vi "Dashboard Main.vi"() -> ()   [LabVIEW 2014]
uses:
  <vilib>/event_ctls.llb/eventvkey.ctl
  <vilib>/Rock Robotics/WPI/Dashboard/WPI_DashboardLogging Global.vi
  <vilib>/Rock Robotics/Network Tables/SD Read Number.vi
  <vilib>/Utility/config.llb/Write Key (String).vi
  <vilib>/Utility/config.llb/Write Key (I32).vi
  <vilib>/Utility/config.llb/NI_LVConfig.lvlib
panel:
  in  "TCP":refnum<k5>
  in  "Rec Mode":enum32{"Stop", "Record", "Playback"}(radio)
  in  "Vision":u16(ring) items=["Camera Off", "USB Camera SW", "USB Camera HW", "IP Camera"]
  out "Camera IP":string
  out "Image Message":string="Timeout in Camera Communications"
  in  "Dashboard Tab":T1(tab)
  in  "Camera Settings":T2={"Frame Rate"=30, "Compression"=30, "Size"=1} {"Frame Rate" scale=1.0..30.0; "Size" items=["640x480", "320x240", "160x120"]}
  out "MotorChart R":cluster{"Numeric":dbl, "Numeric":dbl}(graph)
  out "MotorChart L":T3(graph)
  out "MotorSliders R":cluster{"MotorSlide1":dbl, "MotorSlide2":dbl} {"MotorSlide2" scale=-1.0..1.0 scale format="%#_2e"; "MotorSlide1" scale=-1.0..1.0 scale format="%#_2e"}
  out "MotorSliders L":T4 {"MotorSlide4 2" scale=0.0..14.0 scale format="%#_2e"; "MotorSlide2" scale=-1.0..1.0 scale format="%#_2e"; "MotorSlide1" scale=-1.0..1.0 scale format="%#_2e"}
  out "Gyro":dbl(knob) scale=0.0..360.0
  out "JS1 Z":dbl(slide) scale=-1.0..1.0 scale format="%#_2e"
  out "JS1 Graph":cluster{"X":dbl, "Y":dbl}[](graph)
  out "JS1 Buttons":T5
  out "JS2 Z":dbl(slide) scale=-1.0..1.0 scale format="%#_2e"
  out "JS2 Graph":cluster{"X":dbl, "Y":dbl}[](graph)
  out "JS2 Buttons":T5
  out "Mode":T6(ring)=enum."Auto Disabled"
  in  "DB Camera Config":bool
  out "fps":dbl format="%#.1g"
  out "Mbps":dbl format="%#.1g"
  out "Mbps 2":bool
  in  "DB/String 9":string
  in  "DB/String 8":string
  in  "DB/String 7":string
  in  "DB/String 6":string
  in  "DB/String 5":string
  in  "DB/String 4":string
  in  "DB/String 3":string
  in  "DB/String 2":string
  in  "DB/String 1":string
  in  "DB/String 0":string
  in  "DB/Slider 0":dbl(slide) scale=0.0..5.0
  in  "DB/Slider 1":dbl(slide) scale=0.0..5.0
  in  "DB/Slider 2":dbl(slide) scale=0.0..5.0
  in  "DB/Slider 3":dbl(slide) scale=0.0..5.0
  out "DB/LED 3":bool
  out "DB/LED 2":bool
  out "DB/LED 1":bool
  out "DB/LED 0":bool
  in  "DB/Button 3":bool
  in  "DB/Button 2":bool
  in  "DB/Button 1":bool
  in  "DB/Button 0":bool caption="New Name"
  in  "Autonomous_Modes":bool[](array[boolean])
  in  "Test_Knob":u16(knob) scale=0.0..5.0
  in  "Test Slider":dbl(slide) scale=0.0..100.0 scale format="%#_3g"
  in  "On/Off":bool caption="Solenoid"
  in  "Test Name":u16(ring) items=["Select the test to run...", "Example Test", "-------------------------------", "List of tests is built in robot code.", "Replace with your own automated tests."]
  in  "Test Tree":string(tree)
  in  "Motor":cluster{"Value":dbl, "Enable":bool} {"Value" scale=-1.0..1.0 scale format="%#_3g"}
  out "Progress":T7 {"Test Progress" scale=0.0..100.0}
  in  "Rev/Fwd":cluster{"Forward":bool, "Reverse":bool}
  in  "Test Ring":u16(ring) items=["Monochrome", "Color"]
  in  "Listbox":i32(listbox)
  out "Tree":string(tree)
  out "Camera Image":T8(plugin-control)
  out "Boolean":bool
  # "Left"
  # "Front"
  # "Right"
  # "Battery"
  # "Single Tote"
  # "Double Tote"
  # "Triple Tote"
  # "Butterfly"
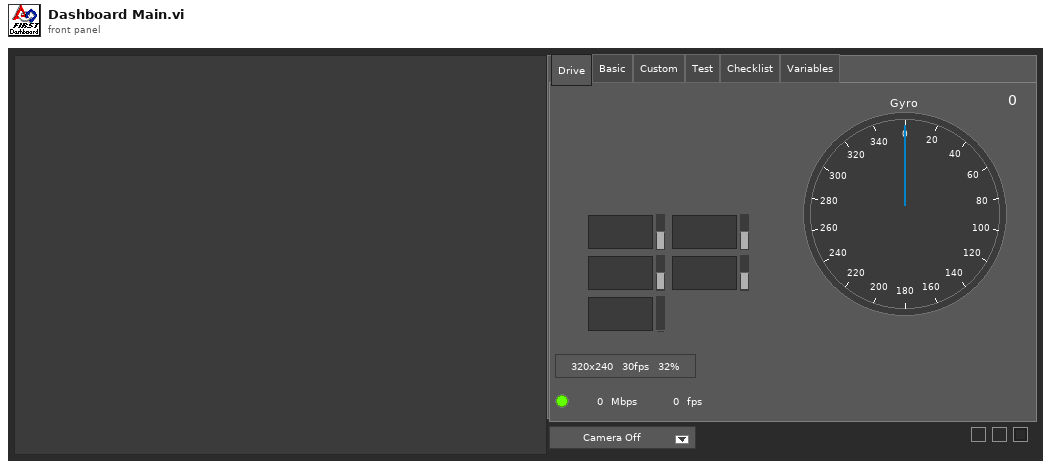
[diagram p1: front panel]
types:
  T1 = enum32{"Drive", "Basic", "Custom", "Test", "Checklist", "Variables"}
  T2 = cluster{"Frame Rate":i32, "Compression":i32, "Size":u16}
  T3 = cluster{"Numeric":dbl, "Numeric":dbl, "Battery V":dbl}
  T4 = cluster{"MotorSlide1":dbl, "MotorSlide2":dbl, "MotorSlide4 2":dbl}
  T5 = cluster{bool, bool, bool, bool, bool, bool, bool, bool, bool, bool, bool, bool}
  T6 = enum8{"Tele-Op Disabled", "Tele-Op Enabled", "Auto Disabled", "Auto Enabled", "Test Disabled", "Test Enabled", "Disconnected", "No Code", "E-Stop"}
  T7 = cluster{"Test Progress":u8, "Test Progress Text":string}
  T8 = typedef "IMAQ Image.ctl" = refnum<image>
  T9 = typedef "Image Type" = u32
  T10 = cluster{"Camera Image":refnum<vi>, "Dashboard Tab":refnum<vi>, "Boolean":refnum<vi>, "Vision":refnum<vi>, "Rec Mode":refnum<vi>, "Test Slider":refnum<vi>, "On/Off ":refnum<vi>, "Test Ring":refnum<vi>, "Rev/Fwd":refnum<vi>, "Test Name":refnum<vi>, "Motor":refnum<vi>, "Progress":refnum<vi>, "CheckList":refnum<vi>, "Tree":refnum<vi>, "Test Tree":refnum<vi>}
  T11 = cluster{"Error Strings":string, "Disable Counts":cluster{u16, u16}, "Rail Faults":cluster{u16, u16, u16}, "Robot IP":string, "DB Mode":u8, "Event Info":cluster{"Name":string, "Type":u8, "Number":u16, "Replay":u8}, "Camera Addr":string}
  T12 = cluster{"Storage":cluster{"Disk Free":u64, "RAM Block":u32, "RAM free":u32}, "CPU Utilization":cluster{"CPU % ISR":sgl, "CPU % Time Crit":sgl, "CPU % Timed Str":sgl, "CPU % High":sgl, "CPU % Above":sgl, "CPU % Normal":sgl, "CPU % Low":sgl}, "CAN":cluster{"% Bus Utilization":sgl, "Bus Off Cnt":u32, "TX_FIFO Full Cnt":u32, "Receive Error Cnt":u8, "Transmit Error Cnt":u8}, "HID":cluster{"HID Outputs":u32, "Rumble Low":u16, "Rumble High":u16}[]}
  T13 = cluster{"Status bits":cluster{"Test Mode":bool, "Autonomous":bool, "Enabled":bool, "Code Start":bool, "Brownout":bool, "Reserved 2":bool, "Reserved 3":bool, "E-Stop":bool}, "Code Trace":cluster{"Disabled":bool, "TeleOp":bool, "Auto":bool, "Test":bool}, "Controller Type":enum16{"unknown", "cRIO", "roboRio"}, "Code?":enum16{"unknown", "noCode", "code"}, "Battery V":dbl}
  T14 = cluster{"Control Bits":cluster{"TestMode":bool, "Autonomous":bool, "Enabled":bool, "FMS Present":bool, bool, bool, bool, "E-Stop":bool}, "Team Station ":u8, "Countdown":sgl, "Joystick Values":cluster{"Axes":dbl[], "Buttons":bool[], "POVs":i16[]}[]}
  T15 = cluster{"Axes":dbl[], "Buttons":bool[], "POVs":i16[]}[]
  T16 = cluster{"Axes":dbl[], "Buttons":bool[], "POVs":i16[]}
  T17 = cluster{"Buttons[0]":bool, "Buttons[1]":bool, "Buttons[2]":bool, "Buttons[3]":bool, "Buttons[4]":bool, "Buttons[5]":bool, "Buttons[6]":bool, "Buttons[7]":bool, "Buttons[8]":bool, "Buttons[9]":bool, "Buttons[10]":bool, "Buttons[11]":bool}
  T18 = typedef "NI_LVConfig.lvlib/Config Data RefNum.ctl" = refnum<k1>
  T19 = cluster{"Operation":enum16{"Update", "Clear"}, "Color Box":u32}[]
  T20 = typedef "eventvkey.ctl" = enum16{"ASCII", "Enter", "Return", "Shift", "Ctrl", "Alt", "Cmd", "Opt", "Caps", "NumLock", "Clear", "Break", "Up", "Down", "Left", "Right", "Insert", "Delete", "Home", "End", "PageUp", "PageDown", "Escape", "Help", "Pause", "ScrollLock", "F1", "F2", "F3", "F4", "F5", "F6", "F7", "F8", "F9", "F10", "F11", "F12", "F13", "F14", "F15", "F16", "F17", "F18", "F19", "F20", "F21", "F22", "F23", "F24", "Play", "VolumeUp", "VolumeDown", "Mute", "Two Byte Char"}
  T21 = cluster{"Image Size":bool, "Image Type":bool, "Pixel Value":bool, "ROI Information":bool, "Zoom Factor":bool}
  T22 = enum8{"Enabled", "Disabled", "Disabled and Grayed Out"}
  T23 = cluster{"Operation":enum16{"Update", "Clear"}, "Color Box":u32}
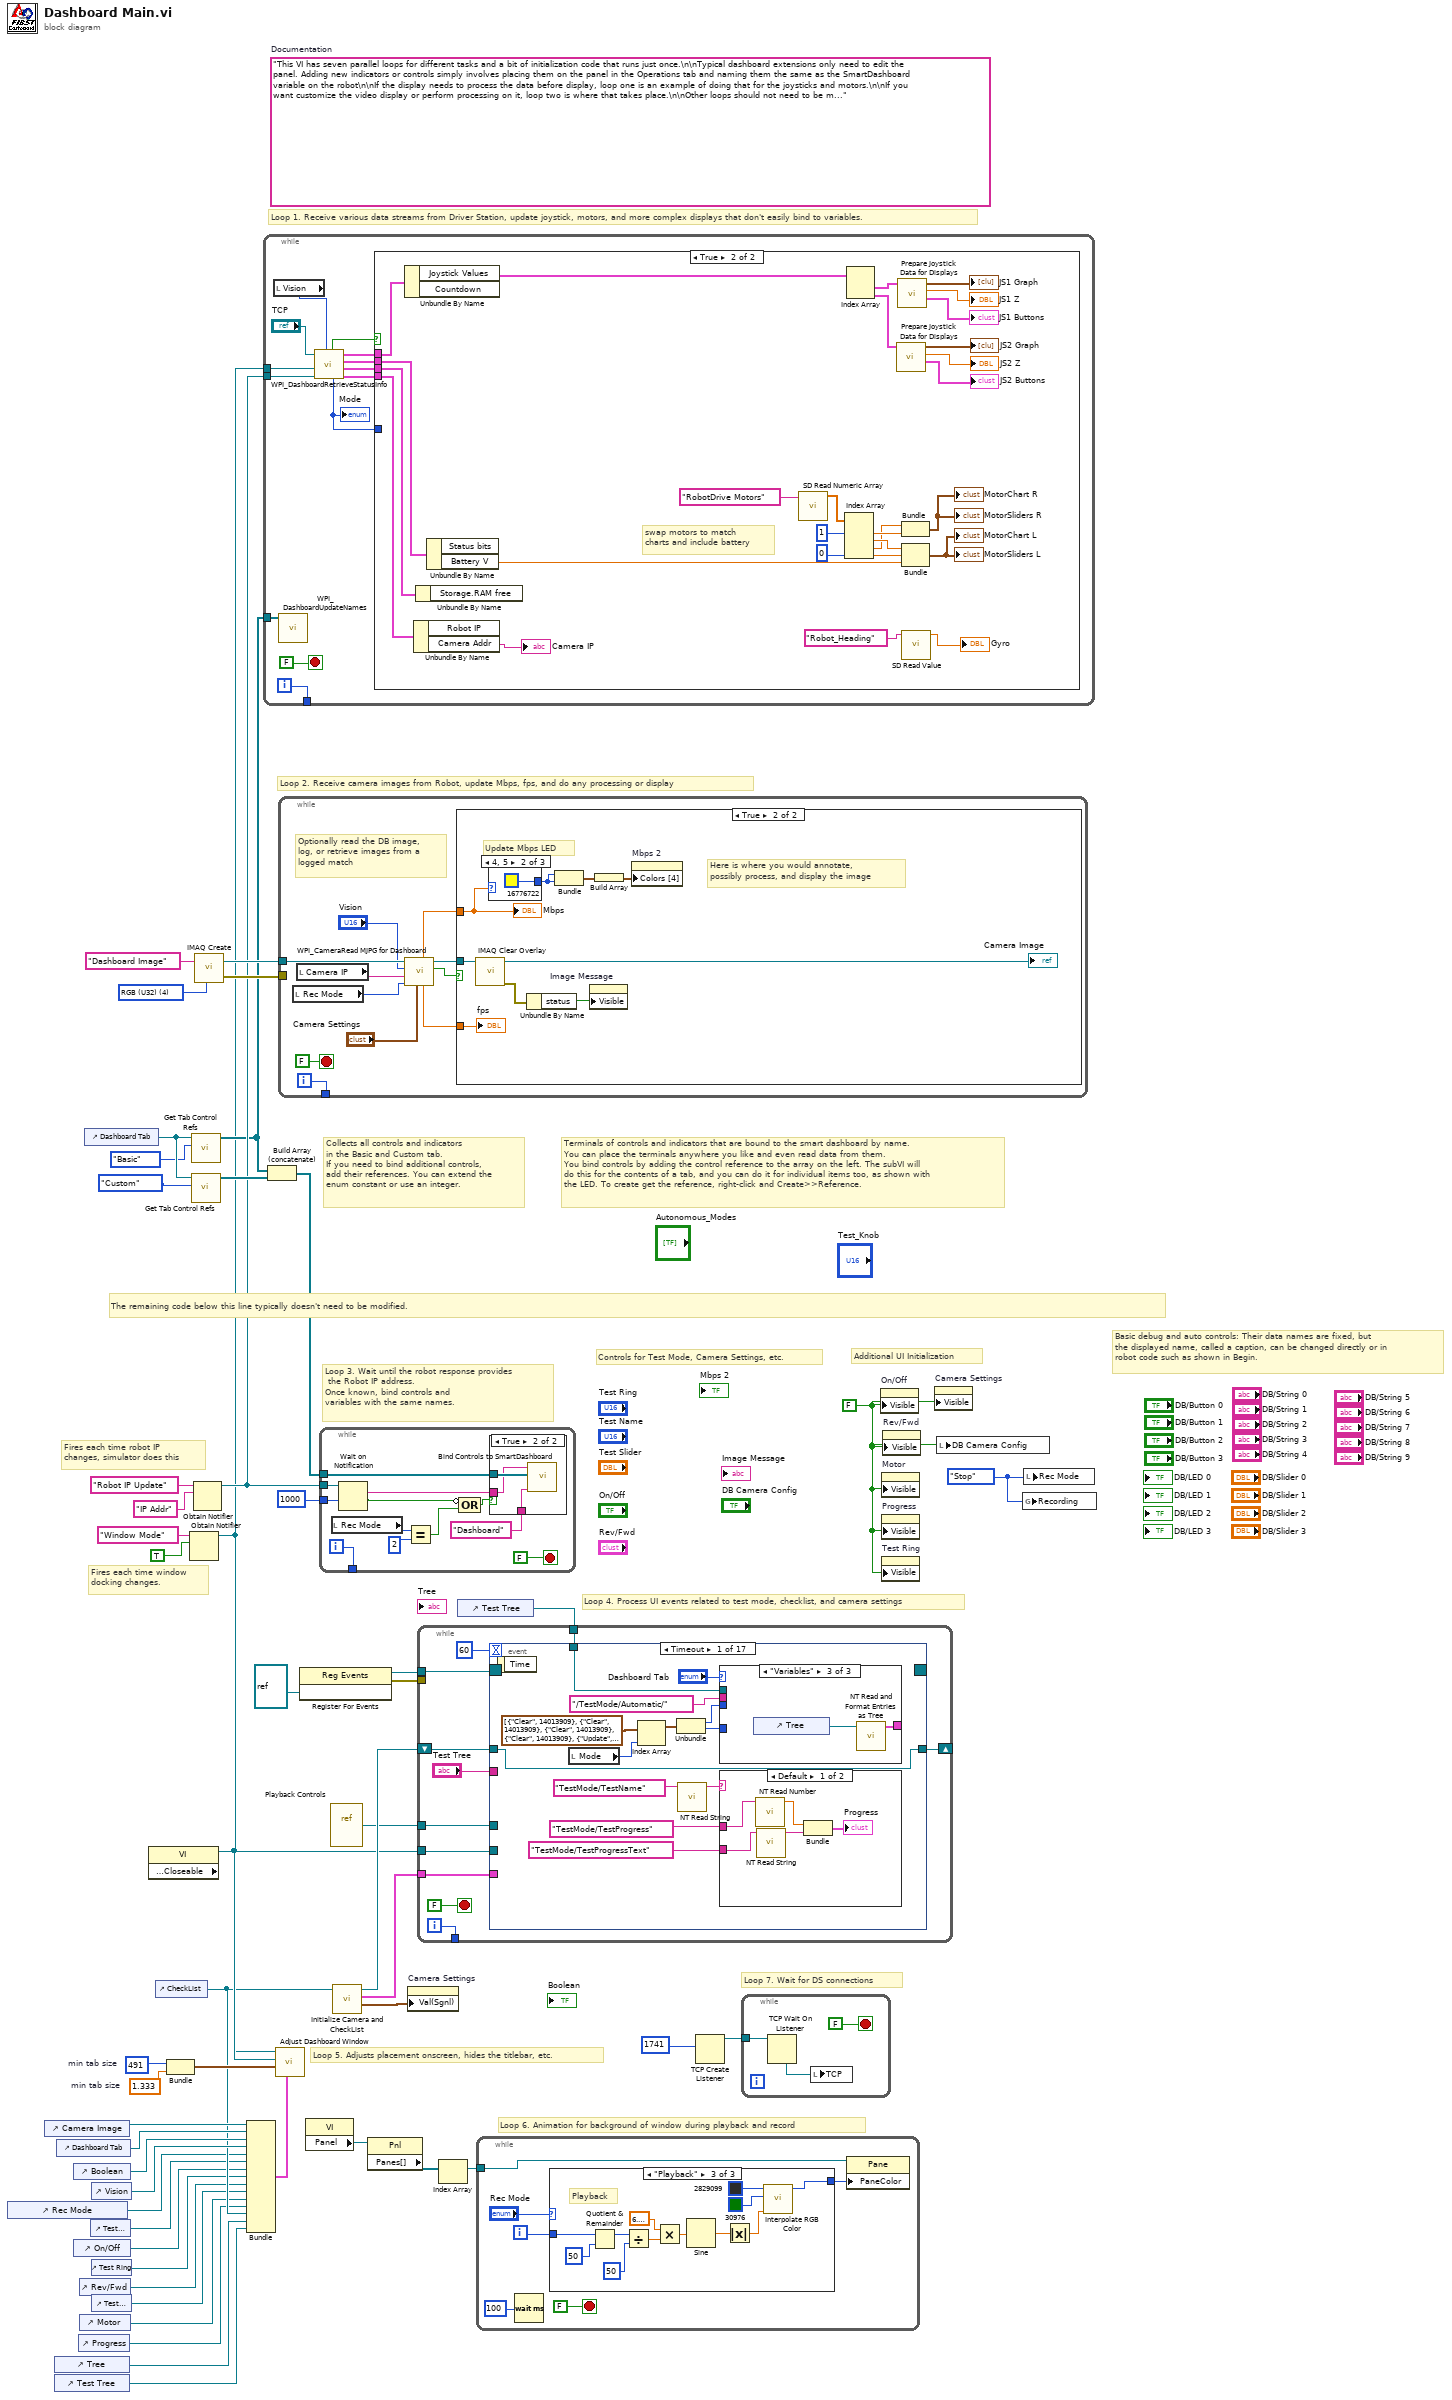
[diagram p0: block diagram]
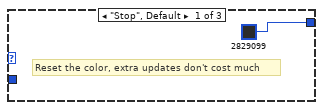
[diagram p3: hidden frame]
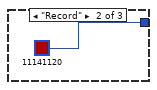
[diagram p4: hidden frame]
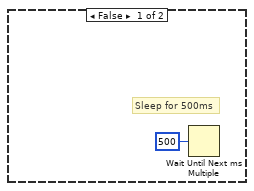
[diagram p6: hidden frame]
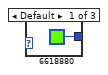
[diagram p7: hidden frame]
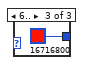
[diagram p8: hidden frame]
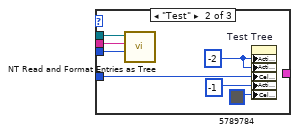
[diagram p10: hidden frame]
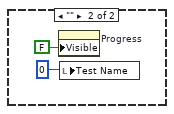
[diagram p11: hidden frame]
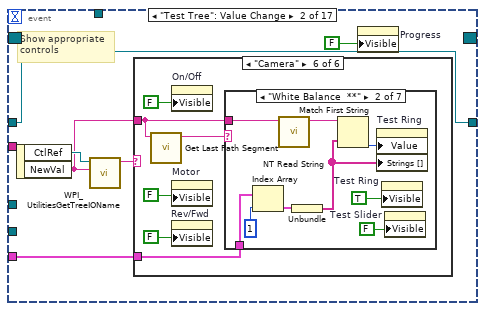
[diagram p12: hidden frame]
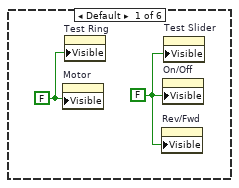
[diagram p13: hidden frame]
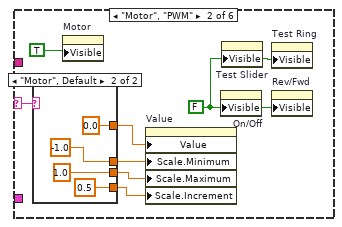
[diagram p14: hidden frame]
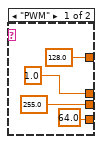
[diagram p15: hidden frame]
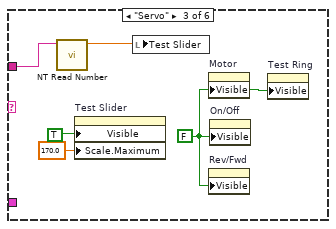
[diagram p16: hidden frame]
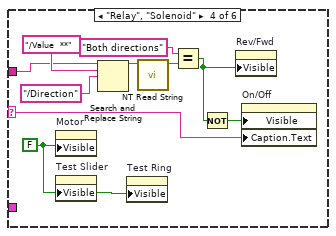
[diagram p17: hidden frame]
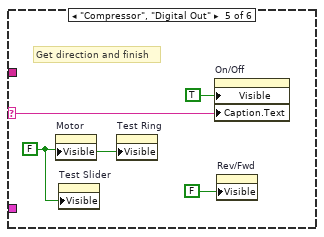
[diagram p18: hidden frame]
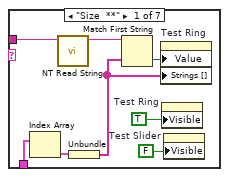
[diagram p19: hidden frame]
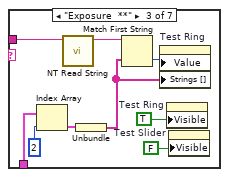
[diagram p20: hidden frame]
diagram:
  w24 = 491  # min tab size
  w23 = 1.333  # min tab size
  w32 = enum32{"Stop", "Record", "Playback"}."Stop" ("Rec Mode")
  w6 = FALSE ("Visible")
  (unwired) "This VI has seven parallel loops for different tasks and a bit of initialization code that runs just once.\n\nTypical dashboard extensions only need to edit the panel. Adding new indicators or controls simply involves placing them on the panel in the Operations tab and naming them the same as the SmartDashboard variable on the robot\n\nIf the display needs to process the data before display, loop one is an example of doing that for the joysticks and motors.\n\nIf you want customize the video display or perform processing on it, loop two is where that takes place.\n\nOther loops should not need to be modified. They are pretty standard, and document the task they perform."  # Documentation
  w52 = T9 4 items=["Grayscale (U8)", "Grayscale (I16)", "Grayscale (SGL)", "Complex (CSG)", "RGB (U32)", "HSL (U32)", "RGB (U64)"] ("Image Type")
  # "Loop 7. Wait for DS connections"
  # "Basic debug and auto controls: Their data names are fixed, but\nthe displayed name, called a caption, can be changed directly or in\nrobot code such as shown in Begin."
  # "Controls for Test Mode, Camera Settings, etc."
  # "Additional UI Initialization"
  # "Loop 6. Animation for background of window during playback and record"
  # "Fires each time robot IP\nchanges, simulator does this"
  # "Fires each time window\ndocking changes."
  # "Collects all controls and indicators\nin the Basic and Custom tab.\nIf you need to bind additional controls,\nadd their references. You can extend the\nenum constant or use an integer."
  # "The remaining code below this line typically doesn't need to be modified."
  # "Loop 4. Process UI events related to test mode, checklist, and camera settings"
  # "Terminals of controls and indicators that are bound to the smart dashboard by name.\nYou can place the terminals anywhere you like and even read data from them.\nYou bind controls by adding the control reference to the array on the left. The subVI will\ndo this for the contents of a tab, and you can do it for individual items too, as shown with\nthe LED. To create get the reference, right-click and Create>>Reference."
  # "Loop 3. Wait until the robot response provides\n the Robot IP address.\nOnce known, bind controls and\nvariables with the same names."
  # "Loop 5. Adjusts placement onscreen, hides the titlebar, etc."
  # "Loop 1. Receive various data streams from Driver Station, update joystick, motors, and more complex displays that don't easily bind to variables."
  # "Loop 2. Receive camera images from Robot, update Mbps, fps, and do any processing or display"
  n1 = control-ref of="Rec Mode"() -> (w12:refnum<vi>)
  n2 = control-ref of="Camera Image"() -> (w27:refnum<vi>)
  n3 = control-ref of="Tree"() -> (w16:refnum<vi>)
  n4 = control-ref of="Test Tree"() -> (w15:refnum<vi>)
  n5 = control-ref of="Dashboard Tab"() -> (w26:refnum<vi>)
  n6 = control-ref of="Boolean"() -> (w21:refnum<vi>)
  n7 = control-ref of="On/Off"() -> (w10:refnum<vi>)
  n8 = control-ref of="Progress"() -> (w7:refnum<vi>)
  n9 = control-ref of="Rev/Fwd"() -> (w8:refnum<vi>)
  n10 = control-ref of="Motor"() -> (w13:refnum<vi>)
  n11 = control-ref of="Dashboard Tab"() -> (w30:refnum<vi>)
  n12 = control-ref of="Test Slider"() -> (w11:refnum<vi>)
  n13 = control-ref of="Vision"() -> (w25:refnum<vi>)
  n14 = control-ref of="Test Ring"() -> (w9:refnum<vi>)
  n15 = control-ref of="Test Name"() -> (w14:refnum<vi>)
  n16 = property class="VI" props=["Front Panel.Closeable"]() -> (reference out=w31:refnum<vi>)  [unwired: 2 in, 2 out]
  n17 = control-ref of="CheckList"() -> (w17:refnum<vi>)
  n18 = Bundle("min tab size"=w24, "min tab size"=w23) -> (w22:cluster{"min tab size":i32, "min tab size":dbl})  [unwired: 1 in]
  n19 = Obtain Notifier(name (unnamed)="Window Mode", notification data type=TRUE) -> (notifier out=w3:refnum<notifier>)  [unwired: 2 in, 2 out]
  n20 = call <vilib>:"Get Tab Control Refs.vi"("Page Index"=T1."Basic" ("Dashboard Tab"), "TabControl in"=w30) -> ("ControlsOnPage"=w4:refnum<vi>[])  [unwired: 9 in]
  n21 = call <vilib>:"Get Tab Control Refs.vi"("Page Index"=T1."Custom" ("Dashboard Tab"), "TabControl in"=w30) -> ("ControlsOnPage"=w29:refnum<vi>[])  [unwired: 9 in]
  n22 = Obtain Notifier(name (unnamed)="Robot IP Update", notification data type="IP Addr" ("name (unnamed)")) -> (notifier out=w5:refnum<notifier>)  [unwired: 2 in, 2 out]
  n23 = call "IMAQ Create"("Image Name"="Dashboard Image", "Image Type"=w52) -> ("New Image"=w50:T8, "error out"=w49:errorcluster)  [unwired: 2 in, 1 out]
  n24 = Bundle("Camera Image"=w27, "Dashboard Tab"=w26, "Boolean"=w21, "Vision"=w25, "Rec Mode"=w12, "Test Slider"=w11, "On/Off"=w10, "Test Ring"=w9, "Rev/Fwd"=w8, "Test Name"=w14, "Motor"=w13, "Progress"=w7, "CheckList"=w17, "Tree"=w16, "Test Tree"=w15) -> (w18:T10)  [unwired: 1 in]
  n25 = while {
    tunnel: [w64] -> _
    tunnel: w5 -> [w58]
    tunnel: w4 -> [w57]
    tunnel: w3 -> [w53]
    i -> [w64]
    stop <- FALSE stop-if-true
    n26 = local read "Vision"() -> (w55:u16)
    n27 = call <vilib>:"WPI_DashboardUpdateNames.vi"("Controls on Tab"=w57) -> ()  [unwired: 11 in]
    n28 = call <vilib>:"WPI_DashboardRetrieveStatusInfo.vi"("Vision"=w55, "Binding Refnum"=w58, "Window Mode Notifier"=w53, "TCP Cnx"="TCP") -> ("Power and Errors"=w59:T11, "Robot Metrics"=w62:T12, "Status Info"=w63:T13, "Control Info"=w60:T14, "Robot Mode"=w56:T6, "Process?"=w61:bool)  [unwired: 2 in]
    "Mode" <- w56
    n29 = case shown="True" w61 {
      tunnel: w63 -> [_ w92]
      tunnel: w62 -> [_ w91]
      tunnel: w60 -> [_ w90]
      tunnel: w59 -> [_ w89]
      tunnel: w56 -> [_ _]
      frame False {
      }
      frame True {
        # "swap motors to match\ncharts and include battery"
        n30 = Unbundle By Name(w90) -> ("Joystick Values"=w77:T15)  [unwired: 1 out]
        n31 = Unbundle By Name(w89) -> ("Camera Addr"=→"Camera IP":string)  [unwired: 1 out]
        n32 = Unbundle By Name(w91) -> ()  [unwired: 1 out]
        n33 = Unbundle By Name(w92) -> ("Battery V"=w78:dbl)  [unwired: 1 out]
        n34 = call <vilib>:"SD Read Numeric Array.vi"("Name"="RobotDrive Motors") -> ("Numeric Array"=w80:dbl[])  [unwired: 8 in, 2 out]
        n35 = Index Array(array=w80, index #1=1, index #4=0) -> (element #1=w84:dbl, element #2=w85:dbl, element #3=w83:dbl, element #4=w88:dbl)  [unwired: 2 in]
        n36 = Index Array(array=w77) -> (element #1=w76:T16, element #2=w71:T16)  [unwired: 2 in]
        n37 = call "Prepare Joystick Data for Displays.vi"("Joystick Values"=w71) -> ("Buttons"=→"JS2 Buttons":T17, "Z Axis"=→"JS2 Z":dbl, "Cartesian Data"=→"JS2 Graph":cluster{"X axis":dbl, "X axis":dbl}[])  [unwired: 8 in]
        n38 = call "Prepare Joystick Data for Displays.vi"("Joystick Values"=w76) -> ("Buttons"=→"JS1 Buttons":T17, "Z Axis"=→"JS1 Z":dbl, "Cartesian Data"=→"JS1 Graph":cluster{"X axis":dbl, "X axis":dbl}[])  [unwired: 8 in]
        n39 = Bundle("Numeric"=w83, "Numeric"=w84) -> (→"MotorChart R" →"MotorSliders R":cluster{"Numeric":dbl, "Numeric":dbl})  [unwired: 1 in]
        n40 = Bundle("Numeric"=w85, "Numeric"=w88, "Battery V"=w78) -> (→"MotorChart L" →"MotorSliders L":T3)  [unwired: 1 in]
        n41 = call-poly <vilib>:"SD Read Value.vi"("Name"="Robot_Heading") -> ("Numeric"=→"Gyro":dbl)  [unwired: 8 in, 2 out]
      }
    }
  }
  n42 = Build Array (concatenate)(w4, w29) -> (w28:refnum<vi>[])
  n43 = call "Adjust Dashboard Window.vi"("Sizing Refnums"=w18, "Size Constraints"=w22, "VI"=w31, "Notifier in"=w3) -> ()  [unwired: 8 in]
  n44 = while {
    tunnel: w50 -> [w101]
    tunnel: w49 -> [_]
    tunnel: [w102] -> _
    i -> [w102]
    stop <- FALSE stop-if-true
    # "Optionally read the DB image,\nlog, or retrieve images from a\nlogged match"
    n45 = local read "Rec Mode"() -> (w95:enum32{"Stop", "Record", "Playback"})
    n46 = local read "Camera IP"() -> (w93:string)
    n47 = call <vilib>:"WPI_CameraRead MJPG for Dashboard.vi"("Camera Settings"="Camera Settings", "Rec Mode"=w95, "Camera IP"=w93, "Camera Mode"="Vision", "Refnum in"=w101) -> ("Active"=w99:bool, "Refnum out"=w100:T8, "FPS"=w98:dbl, "Bandwidth (Mbps)"=w97:dbl)  [unwired: 3 in]
    n48 = case shown="True" w99 {
      tunnel: w100 -> [_ w108]
      tunnel: w97 -> [_ w107]
      tunnel: w98 -> [_ w105]
      frame False {
        # "Sleep for 500ms"
        n49 = Wait Until Next ms Multiple(millisecond multiple=u32 500) -> ()  [unwired: 1 out]
      }
      frame True {
        # "Here is where you would annotate,\npossibly process, and display the image"
        # "Update Mbps LED"
        n50 = call "IMAQ Clear Overlay"("Image"=w108) -> ("error out"=w112:errorcluster, "Image Out"=→"Camera Image":T8)  [unwired: 2 in, 7 out]
        n51 = case shown="4, 5" w107 {
          tunnel: [u32 6618880 ("Color Box") u32 16776722 ("Color Box") u32 16716800 ("Color Box")] -> w109
          frame Default {
          }
          frame 4, 5 {
          }
          frame 6.. {
          }
        }
        n52 = Unbundle By Name(w112) -> ("status"=w113:bool)
        n53 = Bundle("Color Box"=w109, "Color Box"=w109) -> (w111:cluster{"Color Box":u32, "Color Box":u32})  [unwired: 1 out]
        n54 = property on="Image Message" class="Str"("Visible"=w113) -> ()  [unwired: 2 in, 2 out]
        n55 = Build Array(w111) -> (w110:cluster{"Color Box":u32, "Color Box":u32}[])
        n56 = property on="Mbps 2" class="Bool (strict)"("Colors [4]"=w110) -> ()  [unwired: 2 in, 2 out]
        "Mbps" <- w107
        "fps" <- w105
      }
    }
  }
  n57 = register-events(refnum<vi> refnum) -> (reference out=w36:refnum<event-registration>, error out=w35:errorcluster)  [unwired: 2 in]
  n58 = property class="VI"() -> ("Panel"=w39:refnum<vi>)  [unwired: 2 in, 2 out]
  n59 = while {
    tunnel: w28 -> [w128]
    tunnel: w5 -> [w126]
    tunnel: [w124] -> _
    tunnel: u32 1000 ("milliseconds to wait") -> [w123]
    i -> [w124]
    stop <- FALSE stop-if-true
    n60 = local read "Rec Mode"() -> (w119:enum32{"Stop", "Record", "Playback"})
    n61 = Wait on Notification(notifier=w126, timeout in ms (-1)=w123) -> (notification=w125:string, timed out?=w121:bool)  [unwired: 2 in, 2 out]
    n62 = Equal?(x=w119, y=u16 2 ("Rec Mode")) -> (x = y?=w120:bool)
    n63 = Compound Arithmetic op=OR(invert w121, w120) -> (w122:bool)
    n64 = case shown="True" w122 {
      tunnel: w128 -> [_ w131]
      tunnel: w125 -> [_ w130]
      tunnel: "Dashboard" -> [_ w129]
      frame False {
      }
      frame True {
        n65 = call <vilib>:"Bind Controls to SmartDashboard.vi"("Client Name"=w129, "Bound Control Refs"=w131, "Server IP Address"=w130) -> ()  [unwired: 9 in]
      }
    }
  }
  n66 = vi-ref "Playback Controls.vi"() -> (w37:refnum<vi>)
  n67 = call "Initialize Camera and CheckList.vi"("ListBox in"=w17) -> ("Cluster"=w43:cluster{"value":i32, "value":i32, "index":i32}, "Array"=w44:cluster{string[]}[], "File Refnum"=w42:T18)  [unwired: 8 in]
  n68 = property class="Pnl"(reference=w39) -> ("Panes[]"=w40:refnum<vi>[])  [unwired: 1 in, 2 out]
  n69 = property on="Camera Settings" class="Clust (strict)"("Val(Sgnl)"=w43) -> ()  [unwired: 2 in, 2 out]
  n70 = Index Array(array=w40) -> (element=w38:refnum<vi>)  [unwired: 1 in]
  n71 = control-ref of="Test Tree"() -> (w41:refnum<vi>)
  n72 = while {
    tunnel: w44 -> [w139]
    shift-right: [w138] -> _
    shift-left: w42 -> [w137]
    tunnel: [w136] -> _
    tunnel: w41 -> [w135]
    tunnel: w37 -> [w134]
    tunnel: w36 -> [w133]
    tunnel: w35 -> [_]
    tunnel: w31 -> [w132]
    i -> [w136]
    stop <- FALSE stop-if-true
    n73 = event shown="[0] Timeout" {
      selector: w133 -> [_ _ _ _ _ _ _ _ _ _ _ _ _ _ _ _ _]
      dyn-events: [_ _ _ _ _ _ _ _ _ _ _ _ _ w377 _ _ _] -> _
      timeout: u32 60 ("milliseconds to wait") -> [_ _ _ _ _ _ _ _ _ _ _ _ _ _ _ _ _]
      tunnel: w135 -> [w151 _ _ _ _ _ _ _ _ _ _ _ _ _ _ _ _]
      tunnel: "Test Tree" -> [_ _ _ _ _ _ _ _ w346 w354 w356 w360 w368 _ _ _ _]
      tunnel: w139 -> [_ w173 _ _ _ _ w310 w340 _ _ _ _ _ _ _ _ _]
      tunnel: [w147 w172 w271 w276 w284 w296 w309 w333 w345 w352 w355 w359 w367 w379 w393 w394 w404] -> w138
      tunnel: w137 -> [w147 w172 w271 w276 w284 w296 w308 w333 w345 w352 w355 w359 w367 w379 w393 w394 w404]
      tunnel: w134 -> [_ _ _ _ _ _ _ _ _ _ _ _ _ w380 _ w397 _]
      tunnel: w132 -> [_ _ _ _ _ _ _ _ _ _ _ _ _ w375 _ _ _]
      event Timeout {
        n74 = event-data() -> ()  [unwired: 1 in, 1 out]
        n75 = local read "Mode"() -> (w150:T6)
        n76 = Index Array(array=T19 [{"Operation"=enum."Clear", "Color Box"=14013909}, {"Operation"=enum."Clear", "Color Box"=14013909}, {"Operation"=enum."Clear", "Color Box"=14013909}, {"Operation"=enum."Clear", "Color Box"=14013909}, {"Operation"=enum."Update", "Color Box"=14013909}, {"Operation"=enum."Update", "Color Box"=16777215}, {"Operation"=enum."Clear", "Color Box"=14013909}, {"Operation"=enum."Clear", "Color Box"=14013909}, {"Operation"=enum."Clear", "Color Box"=14013909}], index=w150) -> (element=w145:T23)
        n77 = Unbundle(w145) -> ("Operation"=w144:enum16{"Update", "Clear"}, "Color Box"=w143:u32)
        n78 = call <vilib>:"NT Read String.vi"("Name"="TestMode/TestName") -> ("String"=w154:string)  [unwired: 9 in, 1 out]
        n79 = case shown="\"Variables\"" "Dashboard Tab" {
          tunnel: w151 -> [_ w162 _]
          tunnel: "/TestMode/Automatic/" ("Name Pattern") -> [_ w161 _]
          tunnel: w144 -> [_ w160 _]
          tunnel: [_ _ w164] -> _
          tunnel: w143 -> [_ w156 _]
          frame "Custom", Default {
          }
          frame "Test" {
            w159 = -2 ("Active Item:Row Number")
            n80 = call <vilib>:"NT Read and Format Entries as Tree.vi"("Operation"=w160, "Name Pattern"=w161, "Tree Refnum"=w162) -> ()  [unwired: 7 in, 2 out]
            n81 = property on="Test Tree" class="Tree (strict)"("Active Item Row Number"=w159, "ActiveColNum"=w159, "CellBG"=w156, "Active Item Row Number"=-1 ("Active Item:Row Number"), "CellBG"=u32 5789784 ("Color Box")) -> ()  [unwired: 2 in, 2 out]
          }
          frame "Variables" {
            n82 = control-ref of="Tree"() -> (w163:refnum<vi>)
            n83 = call <vilib>:"NT Read and Format Entries as Tree.vi"("Tree Refnum"=w163) -> ("Formatted Strings"=w164:cluster{"Name":string, "Value":string}[])  [unwired: 9 in, 1 out]
          }
        }
        n84 = case shown="Default" w154 {
          tunnel: "TestMode/TestProgress" ("Name") -> [w166 _]
          tunnel: "TestMode/TestProgressText" ("Name") -> [w165 _]
          frame Default {
            n85 = call <vilib>:"NT Read Number.vi"("Name"=w166) -> ("Numeric"=w167:dbl)  [unwired: 9 in, 1 out]
            n86 = call <vilib>:"NT Read String.vi"("Name"=w165) -> ("String"=w168:string)  [unwired: 9 in, 1 out]
            n87 = Bundle("Numeric"=w167, "String"=w168) -> (→"Progress":cluster{"Numeric":dbl, "String":string})  [unwired: 1 in]
          }
          frame "" {
            n88 = property on="Progress" class="Clust (strict)"("Visible"=FALSE) -> ()  [unwired: 2 in, 2 out]
            n89 = local write "Test Name"(u16 0) -> ()
          }
        }
      }
      event "Test Tree": Value Change {
        # "Show appropriate\ncontrols"
        n90 = event-data() -> ("CtlRef"=w176:refnum<vi>, "NewVal"=w174:string)  [unwired: 1 in]
        n91 = call <vilib>:"WPI_UtilitiesGetTreeIOName.vi"("NewVal"=w174, "TreeControl in"=w176) -> ("I/O Name"=w177:string)  [unwired: 9 in]
        n92 = case shown="\"Camera\"" w177 {
          selector: w177 -> [_ w184 _ w202 w211 _]
          tunnel: w174 -> [_ _ w199 w201 _ w218]
          tunnel: w173 -> [_ _ _ _ _ w217]
          frame Default {
            w179 = FALSE ("Visible")
            w178 = FALSE ("Visible")
            n93 = property on="Motor" class="Clust (strict)"("Visible"=w178) -> ()  [unwired: 2 in, 2 out]
            n94 = property on="Test Ring" class="Ring (strict)"("Visible"=w178) -> ()  [unwired: 2 in, 2 out]
            n95 = property on="Rev/Fwd" class="Clust (strict)"("Visible"=w179) -> ()  [unwired: 2 in, 2 out]
            n96 = property on="On/Off" class="Bool (strict)"("Visible"=w179) -> ()  [unwired: 2 in, 2 out]
            n97 = property on="Test Slider" class="Slide (strict)"("Visible"=w179) -> ()  [unwired: 2 in, 2 out]
          }
          frame "Motor", "PWM" {
            w185 = FALSE ("Visible")
            n98 = case shown="\"Motor\", Default" w184 {
              tunnel: [1.0 ("Value") -1.0 ("Value")] -> w183
              tunnel: [255.0 ("Value") 1.0 ("Value")] -> w182
              tunnel: [128.0 ("Value") 0.0 ("Value")] -> w181
              tunnel: [64.0 ("Value") 0.5 ("Value")] -> w180
              frame "PWM" {
              }
              frame "Motor", Default {
              }
            }
            n99 = property on="Motor" class="Clust (strict)"("Visible"=TRUE) -> ()  [unwired: 2 in, 2 out]
            n100 = property on="Value" class="Slide (strict)"("Value"=w181, "Scale.Minimum"=w183, "Scale.Maximum"=w182, "Scale.Increment"=w180) -> ()  [unwired: 2 in, 2 out]
            n101 = property on="On/Off" class="Bool (strict)"("Visible"=w185) -> ()  [unwired: 2 in, 2 out]
            n102 = property on="Test Slider" class="Slide (strict)"("Visible"=w185) -> ()  [unwired: 2 in, 2 out]
            n103 = property on="Test Ring" class="Ring (strict)"("Visible"=w185) -> ()  [unwired: 2 in, 2 out]
            n104 = property on="Rev/Fwd" class="Clust (strict)"("Visible"=w185) -> ()  [unwired: 2 in, 2 out]
          }
          frame "Servo" {
            w197 = FALSE ("Visible")
            n105 = call <vilib>:"NT Read Number.vi"("Name"=w199) -> ("Numeric"=w198:dbl)  [unwired: 9 in, 1 out]
            n106 = property on="Test Slider" class="Slide (strict)"("Visible"=TRUE, "Scale.Maximum"=170.0 ("Scale.Range:Maximum")) -> ()  [unwired: 2 in, 2 out]
            n107 = local write "Test Slider"(w198) -> ()
            n108 = property on="Motor" class="Clust (strict)"("Visible"=w197) -> ()  [unwired: 2 in, 2 out]
            n109 = property on="Rev/Fwd" class="Clust (strict)"("Visible"=w197) -> ()  [unwired: 2 in, 2 out]
            n110 = property on="On/Off" class="Bool (strict)"("Visible"=w197) -> ()  [unwired: 2 in, 2 out]
            n111 = property on="Test Ring" class="Ring (strict)"("Visible"=w197) -> ()  [unwired: 2 in, 2 out]
          }
          frame "Relay", "Solenoid" {
            w200 = FALSE ("Visible")
            n112 = property on="Motor" class="Clust (strict)"("Visible"=w200) -> ()  [unwired: 2 in, 2 out]
            n113 = property on="Test Slider" class="Slide (strict)"("Visible"=w200) -> ()  [unwired: 2 in, 2 out]
            n114 = Search and Replace String(input string=w201, search string="/Value  **", replace string="/Direction") -> (result string=w207:string)  [unwired: 5 in, 3 out]
            n115 = property on="Test Ring" class="Ring (strict)"("Visible"=w200) -> ()  [unwired: 2 in, 2 out]
            n116 = call <vilib>:"NT Read String.vi"("Name"=w207) -> ("String"=w205:string)  [unwired: 9 in, 1 out]
            n117 = Equal?(x="Both directions", y=w205) -> (x = y?=w203:bool)
            n118 = Not(x=w203) -> (.not. x?=w204:bool)
            n119 = property on="Rev/Fwd" class="Clust (strict)"("Visible"=w203) -> ()  [unwired: 2 in, 2 out]
            n120 = property on="On/Off" class="Bool (strict)"("Visible"=w204, "Caption.Text"=w202) -> ()  [unwired: 2 in, 2 out]
          }
          frame "Compressor", "Digital Out" {
            w210 = FALSE ("Visible")
            # "Get direction and finish"
            n121 = property on="Motor" class="Clust (strict)"("Visible"=w210) -> ()  [unwired: 2 in, 2 out]
            n122 = property on="Test Slider" class="Slide (strict)"("Visible"=w210) -> ()  [unwired: 2 in, 2 out]
            n123 = property on="Test Ring" class="Ring (strict)"("Visible"=w210) -> ()  [unwired: 2 in, 2 out]
            n124 = property on="On/Off" class="Bool (strict)"("Visible"=TRUE, "Caption.Text"=w211) -> ()  [unwired: 2 in, 2 out]
            n125 = property on="Rev/Fwd" class="Clust (strict)"("Visible"=FALSE) -> ()  [unwired: 2 in, 2 out]
          }
          frame "Camera" {
            n126 = call <vilib>:"Get Last Path Segment.vi"("String in"=w218) -> ("String out"=w219:string)  [unwired: 10 in]
            n127 = property on="On/Off" class="Bool (strict)"("Visible"=FALSE) -> ()  [unwired: 2 in, 2 out]
            n128 = property on="Motor" class="Clust (strict)"("Visible"=FALSE) -> ()  [unwired: 2 in, 2 out]
            n129 = property on="Rev/Fwd" class="Clust (strict)"("Visible"=FALSE) -> ()  [unwired: 2 in, 2 out]
            n130 = case shown="\"White Balance  **\"" w219 {
              tunnel: w218 -> [w225 w234 w243 w252 w261 _ w267]
              tunnel: w217 -> [w223 w231 w240 w249 w258 _ _]
              frame "Size  **" {
                n131 = Index Array(array=w223) -> (element=w222:cluster{string[]})  [unwired: 1 in]
                n132 = call <vilib>:"NT Read String.vi"("Name"=w225) -> ("String"=w224:string)  [unwired: 9 in, 1 out]
                n133 = Unbundle(w222) -> (w220:string[])
                n134 = Match First String(2:w220, 3:w224) -> (0:w221:i32)  [unwired: 1 out]
                n135 = property on="Test Ring" class="Ring (strict)"("Value"=w221, "Strings []"=w220) -> ()  [unwired: 2 in, 2 out]
                n136 = property on="Test Ring" class="Ring (strict)"("Visible"=TRUE) -> ()  [unwired: 2 in, 2 out]
                n137 = property on="Test Slider" class="Slide (strict)"("Visible"=FALSE) -> ()  [unwired: 2 in, 2 out]
              }
              frame "White Balance  **" {
                n138 = Index Array(array=w231, index=1) -> (element=w232:cluster{string[]})
                n139 = call <vilib>:"NT Read String.vi"("Name"=w234) -> ("String"=w233:string)  [unwired: 9 in, 1 out]
                n140 = Unbundle(w232) -> (w229:string[])
                n141 = Match First String(2:w229, 3:w233) -> (0:w228:i32)  [unwired: 1 out]
                n142 = property on="Test Ring" class="Ring (strict)"("Value"=w228, "Strings []"=w229) -> ()  [unwired: 2 in, 2 out]
                n143 = property on="Test Ring" class="Ring (strict)"("Visible"=TRUE) -> ()  [unwired: 2 in, 2 out]
                n144 = property on="Test Slider" class="Slide (strict)"("Visible"=FALSE) -> ()  [unwired: 2 in, 2 out]
              }
              frame "Exposure  **" {
                n145 = Index Array(array=w240, index=2) -> (element=w241:cluster{string[]})
                n146 = call <vilib>:"NT Read String.vi"("Name"=w243) -> ("String"=w242:string)  [unwired: 9 in, 1 out]
                n147 = Unbundle(w241) -> (w237:string[])
                n148 = Match First String(2:w237, 3:w242) -> (0:w238:i32)  [unwired: 1 out]
                n149 = property on="Test Ring" class="Ring (strict)"("Value"=w238, "Strings []"=w237) -> ()  [unwired: 2 in, 2 out]
                n150 = property on="Test Ring" class="Ring (strict)"("Visible"=TRUE) -> ()  [unwired: 2 in, 2 out]
                n151 = property on="Test Slider" class="Slide (strict)"("Visible"=FALSE) -> ()  [unwired: 2 in, 2 out]
              }
              frame "Exposure Priority  **" {
                n152 = Index Array(array=w249, index=3) -> (element=w250:cluster{string[]})
                n153 = call <vilib>:"NT Read String.vi"("Name"=w252) -> ("String"=w251:string)  [unwired: 9 in, 1 out]
                n154 = Unbundle(w250) -> (w246:string[])
                n155 = Match First String(2:w246, 3:w251) -> (0:w247:i32)  [unwired: 1 out]
                n156 = property on="Test Ring" class="Ring (strict)"("Value"=w247, "Strings []"=w246) -> ()  [unwired: 2 in, 2 out]
                n157 = property on="Test Ring" class="Ring (strict)"("Visible"=TRUE) -> ()  [unwired: 2 in, 2 out]
                n158 = property on="Test Slider" class="Slide (strict)"("Visible"=FALSE) -> ()  [unwired: 2 in, 2 out]
              }
              frame "Color Enable  **" {
                n159 = Index Array(array=w258, index=4) -> (element=w259:cluster{string[]})
                n160 = call <vilib>:"NT Read String.vi"("Name"=w261) -> ("String"=w260:string)  [unwired: 9 in, 1 out]
                n161 = Unbundle(w259) -> (w255:string[])
                n162 = Match First String(2:w255, 3:w260) -> (0:w256:i32)  [unwired: 1 out]
                n163 = property on="Test Ring" class="Ring (strict)"("Value"=w256, "Strings []"=w255) -> ()  [unwired: 2 in, 2 out]
                n164 = property on="Test Ring" class="Ring (strict)"("Visible"=TRUE) -> ()  [unwired: 2 in, 2 out]
                n165 = property on="Test Slider" class="Slide (strict)"("Visible"=FALSE) -> ()  [unwired: 2 in, 2 out]
              }
              frame Default {
                n166 = property on="Test Ring" class="Ring (strict)"("Visible"=FALSE) -> ()  [unwired: 2 in, 2 out]
                n167 = property on="Test Slider" class="Slide (strict)"("Visible"=FALSE) -> ()  [unwired: 2 in, 2 out]
              }
              frame "Brightness  **", "Color Level  **", "Compression  **", "FPS  **", "Sharpness  **" {
                n168 = call <vilib>:"NT Read Number.vi"("Name"=w267) -> ("Numeric"=w266:dbl)  [unwired: 9 in, 1 out]
                n169 = local write "Test Slider"(w266) -> ()
                n170 = property on="Test Slider" class="Slide (strict)"("Visible"=TRUE, "Scale.Maximum"=100.0 ("Scale.Range:Maximum")) -> ()  [unwired: 2 in, 2 out]
                n171 = property on="Test Ring" class="Ring (strict)"("Visible"=FALSE) -> ()  [unwired: 2 in, 2 out]
              }
            }
          }
        }
        n172 = property on="Progress" class="Clust (strict)"("Visible"=FALSE) -> ()  [unwired: 2 in, 2 out]
      }
      event "Test Name": Mouse Enter {
        # "Populate the ring with the list of tests"
        n173 = event-data() -> ()  [unwired: 1 in, 1 out]
        n174 = call <vilib>:"NT Read String Array.vi"("Name"="TestMode/TestList") -> ("String Array"=w275:string[])  [unwired: 9 in, 1 out]
        n175 = Build Array (concatenate)("Select the test to run...", w275) -> (w274:string[])
        n176 = property on="Test Name" class="Ring (strict)"("Strings []"=w274) -> ()  [unwired: 2 in, 2 out]
      }
      event "Test Name": Value Change {
        w277 = FALSE ("Visible")
        # "Tell the robot the test name to run"
        n177 = event-data() -> ("NewVal"=w281:u16)  [unwired: 1 in]
        n178 = property on="Test Name" class="Ring (strict)"() -> ("Strings []"=w282:string[])  [unwired: 2 in, 2 out]
        n179 = local write "Progress"(T7 {"Test Progress"=0, "Test Progress Text"=""} ("Progress")) -> ()
        n180 = Index Array(array=w282, index=w281) -> (element=w280:string)
        n181 = call <vilib>:"NT Write String.vi"("String"=w280, "Name"="TestMode/TestName") -> ()  [unwired: 9 in, 1 out]
        n182 = property on="Progress" class="Clust (strict)"("Visible"=TRUE) -> ()  [unwired: 2 in, 2 out]
        n183 = property on="Motor" class="Clust (strict)"("Visible"=w277) -> ()  [unwired: 2 in, 2 out]
        n184 = property on="Test Slider" class="Slide (strict)"("Visible"=w277) -> ()  [unwired: 2 in, 2 out]
        n185 = property on="On/Off" class="Bool (strict)"("Visible"=w277) -> ()  [unwired: 2 in, 2 out]
        n186 = property on="Rev/Fwd" class="Clust (strict)"("Visible"=w277) -> ()  [unwired: 2 in, 2 out]
        n187 = property on="Test Ring" class="Ring (strict)"("Visible"=w277) -> ()  [unwired: 2 in, 2 out]
      }
      event "Listbox": Double Click {
        # "Shift clears all"
        # "Update symbols on the listbox"
        n188 = event-data() -> ("PlatMods.Shift"=w285:bool, "Row"=w287:i32)  [unwired: 1 in]
        n189 = case shown="True" w285 {
          tunnel: w287 -> [w291 _]
          tunnel: 1 -> [w290 _]
          frame False {
            n190 = property on="Listbox" class="LstBox (strict)"() -> ("Item Symbols"=w289:i32[])  [unwired: 2 in, 2 out]
            n191 = Replace Array Subset(array=w289, new element=w290, index=w291) -> (w288:i32[])
            n192 = property on="Listbox" class="LstBox (strict)"("Item Symbols"=w288) -> ()  [unwired: 2 in, 2 out]
          }
          frame True {
            w292 = 0 ("Top Row")
            n193 = property on="Listbox" class="LstBox (strict)"() -> ("Number of Rows"=w294:u32)  [unwired: 2 in, 2 out]
            n194 = Initialize Array(0, w294) -> (w293:i32[])
            n195 = property on="Listbox" class="LstBox (strict)"("Top Row"=w292, "Value"=w292, "Item Symbols"=w293) -> ()  [unwired: 2 in, 2 out]
          }
        }
      }
      event "Listbox": Key Down {
        # "Update symbols on the listbox\nLeft and right keys check and uncheck"
        n196 = event-data() -> ("VKey"=w298:T20)  [unwired: 1 in]
        n197 = case shown="\"Left\", \"Right\"" w298 {
          selector: w298 -> [w303 _]
          tunnel: eventvkey."Left" ("VKey") -> [w301 _]
          frame "Left", "Right" {
            n198 = Equal?(x=w301, y=w303) -> (x = y?=w302:bool)
            n199 = Select(t=0, s=w302, f=1) -> (s? t:f=w304:i32)
            n200 = property on="Listbox" class="LstBox (strict)"() -> ("Item Symbols"=w307:i32[])  [unwired: 2 in, 2 out]
            n201 = Replace Array Subset(array=w307, new element=w304, index="Listbox") -> (w306:i32[])
            n202 = property on="Listbox" class="LstBox (strict)"("Item Symbols"=w306) -> ()  [unwired: 2 in, 2 out]
          }
          frame Default {
          }
        }
      }
      event "DB Camera Config": Value Change {
        # "Show or hide the cluster of controls, store in ini file"
        n203 = event-data() -> ("NewVal"=w311:bool)  [unwired: 1 in]
        n204 = case shown="False" w311 {
          tunnel: w310 -> [w320 _]
          tunnel: [w313 w331] -> w309
          tunnel: w308 -> [w312 w331]
          frame False {
            w327 = "Camera"
            w330 = FALSE ("Visible")
            n205 = local read "Camera Settings"() -> (w319:T2)
            n206 = Index Array(array=w320) -> (element=w323:cluster{string[]})  [unwired: 1 in]
            n207 = Unbundle(w319) -> ("Frame Rate"=w318:i32, "Compression"=w317:i32, "Size"=w321:u16)
            n208 = Unbundle(w323) -> (w322:string[])
            n209 = Index Array(array=w322, index=w321) -> (element=w316:string)
            n210 = call-poly <vilib>:"Write Key.vi"("section"=w327, "value"=w316, "key"="Size", "refnum"=w312) -> ("refnum out"=w329:T18)  [unwired: 2 in, 5 out]
            n211 = call-poly <vilib>:"Write Key.vi"("section"=w327, "value"=w318, "key"="FrameRate", "refnum"=w329) -> ("refnum out"=w328:T18)  [unwired: 1 in, 6 out]
            n212 = property on="Camera Settings" class="Clust (strict)"("Visible"=w330) -> ()  [unwired: 2 in, 2 out]
            n213 = local write "DB Camera Config"(w330) -> ()
            n214 = call-poly <vilib>:"Write Key.vi"("section"=w327, "value"=w317, "key"="Compression", "refnum"=w328) -> ("refnum out"=w314:T18)  [unwired: 1 in, 6 out]
            n215 = call <vilib>:"Close Config Data.vi"("refnum"=w314) -> ("file path"=w315:path)  [unwired: 2 in, 8 out]
            n216 = call <vilib>:"Open Config Data.vi"("configuration file path"=w315) -> ("refnum"=w313:T18)  [unwired: 8 in, 2 out]
          }
          frame True {
            n217 = property on="Camera Settings" class="Clust (strict)"("Visible"=TRUE) -> ()  [unwired: 2 in, 2 out]
          }
        }
      }
      event "Camera Settings": Value Change {
        # "Update summary string when any elements of DB camera change"
        n218 = event-data() -> ("NewVal"=w344:T2)  [unwired: 1 in]
        n219 = Index Array(array=w340) -> (element=w339:cluster{string[]})  [unwired: 1 in]
        n220 = Unbundle(w344) -> ("Frame Rate"=w335:i32, "Compression"=w334:i32, "Size"=w337:u16)
        n221 = Unbundle(w339) -> (w338:string[])
        n222 = Index Array(array=w338, index=w337) -> (element=w336:string)
        n223 = Format Into String(format string="%s   %dfps   %d%%", w336, w335, w334) -> (resulting string=w341:string)  [unwired: 2 in, 1 out]
        n224 = Build Array(w341) -> (w342:string[])
        n225 = property on="DB Camera Config" class="Bool (strict)"("Strings [4]"=w342) -> ()  [unwired: 2 in, 2 out]
      }
      event "Motor.Enable": Value Change {
        # "When the test mode otor enable helper is set, update that\ntree row item's value"
        n226 = event-data() -> ("NewVal"=w350:bool)  [unwired: 1 in]
        n227 = Unbundle("Motor") -> ("Value"=w349:dbl)  [unwired: 1 out]
        n228 = Select(t=w349, s=w350, f=0.0) -> (s? t:f=w347:dbl)
        n229 = call <vilib>:"NT Write Number.vi"("Numeric"=w347, "Name"=w346) -> ()  [unwired: 9 in, 1 out]
      }
      event "Test Slider": Value Change {
        # "When the test mode slider helper is set, update that\ntree row item's value"
        n230 = event-data() -> ("NewVal"=w353:dbl)  [unwired: 1 in]
        n231 = call <vilib>:"NT Write Number.vi"("Numeric"=w353, "Name"=w354) -> ()  [unwired: 9 in, 1 out]
      }
      event "On/Off": Value Change {
        # "When the test mode on/off helper value is set, update that\ntree row item's value"
        n232 = event-data() -> ("NewVal"=w358:bool)  [unwired: 1 in]
        n233 = Boolean To (0,1)(Boolean=w358) -> (0, 1=w357:i16)
        n234 = call <vilib>:"NT Write Number.vi"("Numeric"=w357, "Name"=w356) -> ()  [unwired: 9 in, 1 out]
      }
      event "Rev/Fwd": Value Change {
        # "When the test mode helper value for relays is set, update that\ntree row item's value"
        n235 = event-data() -> ("NewVal.Forward"=w366:bool, "NewVal.Reverse"=w365:bool)  [unwired: 1 in]
        n236 = Boolean To (0,1)(Boolean=w366) -> (0, 1=w362:i16)
        n237 = Boolean To (0,1)(Boolean=w365) -> (0, 1=w364:i16)
        n238 = Negate(x=w364) -> (-x=w363:i16)
        n239 = Add(x=w362, y=w363) -> (x+y=w361:i16)
        n240 = call <vilib>:"NT Write Number.vi"("Numeric"=w361, "Name"=w360) -> ()  [unwired: 9 in, 1 out]
      }
      event "Test Ring": Value Change {
        # "When a test mode helper value is selected from the ring,\nset the tree item's variable to the string value"
        n241 = event-data() -> ("NewVal"=w370:u16)  [unwired: 1 in]
        n242 = property on="Test Ring" class="Ring (strict)"() -> ("Strings []"=w371:string[])  [unwired: 2 in, 2 out]
        n243 = Index Array(array=w371, index=w370) -> (element=w369:string)
        n244 = call <vilib>:"NT Write String.vi"("String"=w369, "Name"=w368) -> ()  [unwired: 9 in, 1 out]
      }
      event "Rec Mode": Value Change {
        # "Update globals for recording mode and path to read log from.\nClear when logging and let NetworkTables set path for vision to\nuse."
        n245 = event-data() -> ("NewVal"=w381:enum32{"Stop", "Record", "Playback"})  [unwired: 1 in]
        n246 = global write "WPI_DashboardLogging Global.vi" "Logging Filename"(path "") -> ()
        n247 = case shown="\"Playback\"" w381 {
          tunnel: w380 -> [_ w383 w391]
          tunnel: [_ _ w390] -> w377
          tunnel: [_ _ w389] -> _
          tunnel: w375 -> [_ _ w387]
          tunnel: cluster{i32, i32} {-250, 170} -> [_ _ w386]
          tunnel: [_ _ T21 {"Image Size"=TRUE, "Image Type"=TRUE, "Pixel Value"=TRUE, "ROI Information"=TRUE, "Zoom Factor"=FALSE} ("Image Information Shown:All Elements")] -> w373
          tunnel: [_ _ TRUE ("Zoom Factor")] -> w372
          frame Default {
          }
          frame "Stop", "Record" {
            # "Place Window too"
            n248 = invoke class="VI" method="FP.Close"(reference=w383) -> (reference out=w382:refnum<vi>)  [unwired: 2 in, 2 out]
            n249 = invoke class="VI" method="Abort VI"(reference=w382) -> ()  [unwired: 2 in, 3 out]
          }
          frame "Playback" {
            n250 = call "Open Playback Panel.vi"("Offset"=w386, "DB VI Ref"=w387, "Playback in"=w391) -> ("Playback out"=w388:refnum<vi>)  [unwired: 8 in]
            n251 = register-events(w388) -> (reference out=w390:refnum<event-registration>, error out=w389:errorcluster)  [unwired: 2 in]
          }
        }
        n252 = global write "WPI_DashboardLogging Global.vi" "Recording"(w381) -> ()
        n253 = property on="Camera Image" class="ImageControl"("Image Information Shown"=w373, "Image Information Visible"=w372) -> ()  [unwired: 2 in, 2 out]
        n254 = call <vilib>:"WPI_DashboardNT Log FieldName Cache.vi"("Operation"=enum16{"Lookup/Add", "Index", "Clear"}."Clear") -> ()  [unwired: 8 in, 3 out]
      }
      event Panel Close {
        w392 = enum32{"Stop", "Record", "Playback"}."Stop" ("Rec Mode")
        # "Playback window has been closed, abort"
        n255 = event-data() -> ()  [unwired: 1 in, 4 out]
        n256 = local write "Rec Mode"(w392) -> ()
        n257 = global write "WPI_DashboardLogging Global.vi" "Recording"(w392) -> ()
      }
      event Panel Close {
        # "Abort playback window and ourself"
        n258 = event-data() -> ()  [unwired: 1 in, 4 out]
        n259 = invoke class="VI" method="FP.Close"(reference=w397) -> (reference out=w396:refnum<vi>)  [unwired: 2 in, 2 out]
        n260 = invoke class="VI" method="Abort VI"(reference=w396) -> (error out=w395:errorcluster)  [unwired: 2 in, 2 out]
        n261 = invoke class="VI" method="Abort VI"(error in=w395) -> ()  [unwired: 2 in, 3 out]
      }
      event "Vision": Value Change {
        # "Enable/Disable Compression slider.\nHW USB is hard-coded into the camera"
        n262 = event-data() -> ("NewVal"=w403:u16)  [unwired: 1 in]
        n263 = Equal?(x=w403, y=u32 2 ("milliseconds to wait")) -> (x = y?=w401:bool)
        n264 = Select(t=T22."Disabled and Grayed Out" ("Disabled"), s=w401, f=T22."Enabled" ("Disabled")) -> (s? t:f=w398:T22)
        n265 = property on="Compression" class="Slide (strict)"("DisabledEnum"=w398) -> ()  [unwired: 2 in, 2 out]
      }
    }
  }
  n266 = while {
    tunnel: w38 -> [w406]
    i -> [w409]
    stop <- FALSE stop-if-true
    n267 = Wait (ms)(milliseconds to wait=u32 100) -> ()  [unwired: 1 out]
    n268 = case shown="\"Playback\"" "Rec Mode" {
      tunnel: w409 -> [_ _ w424]
      tunnel: [u32 2829099 ("Base Color") u32 11141120 ("Target Color") w413] -> w405
      frame "Stop", Default {
        # "Reset the color, extra updates don't cost much"
      }
      frame "Record" {
      }
      frame "Playback" {
        # "Playback"
        n269 = Quotient & Remainder(x=w424, y=u32 50 ("milliseconds to wait")) -> (x-y*floor(x/y)=w420:u32)  [unwired: 1 out]
        n270 = Divide(x=w420, y=u32 50 ("milliseconds to wait")) -> (x/y=w417:dbl)
        n271 = Multiply(x=6.283185307179586, y=w417) -> (x*y=w422:dbl)
        n272 = Sine(x=w422) -> (sin(x)=w421:dbl)
        n273 = Absolute Value(x=w421) -> (abs(x)=w414:dbl)
        n274 = call "Interpolate RGB Color.vi"("Proportion"=w414, "Target Color"=u32 30976, "Base Color"=u32 2829099) -> ("Result Color"=w413:u32)  [unwired: 8 in]
      }
    }
    n275 = property class="Pane"(reference=w406, "PaneColor"=w405) -> ()  [unwired: 1 in, 2 out]
  }
  n276 = TCP Create Listener(10:u16 1741 ("timeout ms (25000)")) -> (3:w1:refnum<k5>)  [unwired: 4 in, 2 out]
  n277 = while {
    tunnel: w1 -> [w426]
    stop <- FALSE stop-if-true
    n278 = TCP Wait On Listener(11:w426) -> (4:w425:refnum<k5>)  [unwired: 3 in, 4 out]
    n279 = local write "TCP"(w425) -> ()
  }
  n280 = property on="On/Off" class="Bool (strict)"("Visible"=w6) -> ()  [unwired: 2 in, 2 out]
  n281 = property on="Motor" class="Clust (strict)"("Visible"=w6) -> ()  [unwired: 2 in, 2 out]
  n282 = property on="Progress" class="Clust (strict)"("Visible"=w6) -> ()  [unwired: 2 in, 2 out]
  n283 = property on="Test Ring" class="Ring (strict)"("Visible"=w6) -> ()  [unwired: 2 in, 2 out]
  n284 = property on="Rev/Fwd" class="Clust (strict)"("Visible"=w6) -> ()  [unwired: 2 in, 2 out]
  n285 = property on="Camera Settings" class="Clust (strict)"("Visible"=w6) -> ()  [unwired: 2 in, 2 out]
  n286 = local write "DB Camera Config"(w6) -> ()
  n287 = global write "WPI_DashboardLogging Global.vi" "Recording"(w32) -> ()
  n288 = local write "Rec Mode"(w32) -> ()
